vi "Config Dev Auto.vi"(8 "error in":errorcluster, 9 "Loss (off)":enum16{"off", "on"}(ring), 10 "Capacitance (off)":enum16{"off", "on"}(ring), 11 "VISA resource name":refnum<visa-resource-name>) -> (0 "error out":errorcluster, 3 "VISA resource name out":refnum<visa-resource-name>)   [LabVIEW 2019, in "Andeen-Hagerling 2700(400 firmware).lvlib"]
doc: "Provides settings that determine whether or not a new BBPoint and new DPoint are automatically established during the initialization of the deviation subsystem. When automatic set point generation is enabled for capacitance and/or loss then BBPoint is set equal to the corresponding Initial Deviation Reading when the DEV ON command is executed."
uses:
  Andeen-Hagerling 2700(400 firmware).lvlib
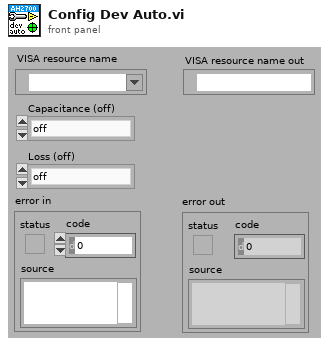
[diagram p1: front panel]
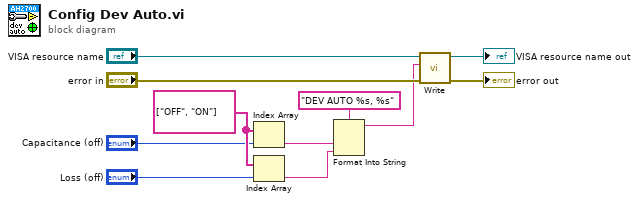
[diagram p0: block diagram]
diagram:
  w5 = string[] ["OFF", "ON"]
  n1 = Index Array(array=w5, index="Capacitance (off)") -> (element=w2:string)
  n2 = Index Array(array=w5, index="Loss (off)") -> (element=w1:string)
  n3 = Format Into String(format string="DEV AUTO %s, %s", w2, w1) -> (resulting string=w6:string)  [unwired: 2 in, 1 out]
  n4 = call "Write.vi"("error in"="error in", "command"=w6, "VISA resource name"="VISA resource name") -> ("error out"=→"error out":errorcluster, "VISA resource name out"=→"VISA resource name out":refnum<visa-resource-name>)  [unwired: 7 in]
